vi "Get Plot at Mouse Click in Legend.vi"(0 "LegNumRows":u32, 5 "Legend:Position":T2, 7 "Legend:Size":T1, 9 "LegScrollPos":u32, 11 "Error In":errorcluster, 12 "Mouse Click Coordinates":cluster{"Horizontal":dbl, "Vertical":dbl}) -> (4 "Click is in Legend?":bool, 8 "Plot Index":i32, 15 "Error Out":errorcluster)   [LabVIEW 2019]
uses:
  <vilib>/Utility/miscctls.llb/LVPositionTypeDef.ctl
  <vilib>/Utility/miscctls.llb/LVBoundsTypeDef.ctl
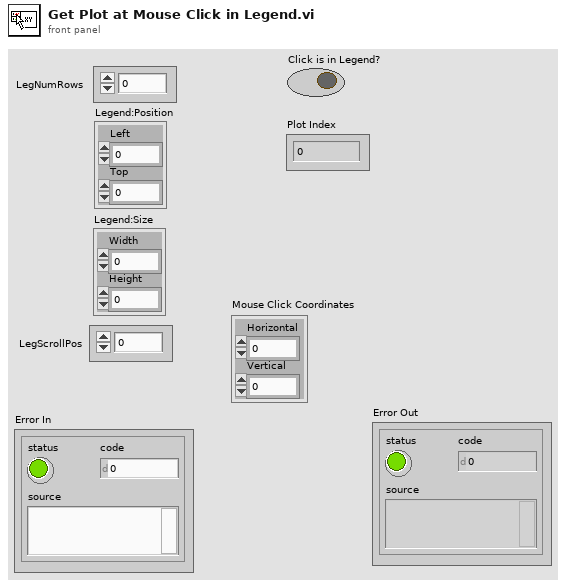
[diagram p1: front panel]
types:
  T1 = typedef "LVBoundsTypeDef.ctl" = cluster{"Width":u32, "Height":u32}
  T2 = typedef "LVPositionTypeDef.ctl" = cluster{"Left":i32, "Top":i32}
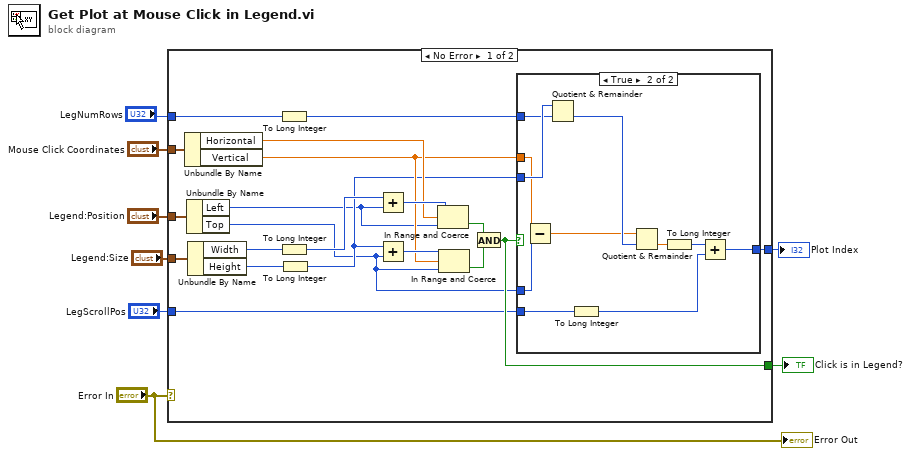
[diagram p0: block diagram]
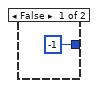
[diagram p2: hidden frame]
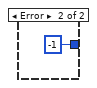
[diagram p3: hidden frame]
diagram:
  n1 = case shown="No Error" "Error In" {
    tunnel: "Mouse Click Coordinates" -> [w24 _]
    tunnel: "LegNumRows" -> [w22 _]
    tunnel: [w20 -1] -> w6
    tunnel: [w19 _] -> w5
    tunnel: "LegScrollPos" -> [w18 _]
    tunnel: "Legend:Position" -> [w14 _]
    tunnel: "Legend:Size" -> [w12 _]
    frame No Error {
      n2 = Unbundle By Name(w24) -> ("Horizontal"=w23:dbl, "Vertical"=w21:dbl)
      n3 = Unbundle By Name(w14) -> ("Left"=w9:i32, "Top"=w13:i32)
      n4 = Unbundle By Name(w12) -> ("Width"=w11:u32, "Height"=w10:u32)
      n5 = To Long Integer(number=w22) -> (32bit integer=w15:i32)
      n6 = To Long Integer(number=w11) -> (32bit integer=w17:i32)
      n7 = To Long Integer(number=w10) -> (32bit integer=w16:i32)
      n8 = Add(x=w17, y=w9) -> (x+y=w25:i32)
      n9 = Add(x=w16, y=w13) -> (x+y=w26:i32)
      n10 = In Range and Coerce(upper limit=w25, x=w23, lower limit=w9) -> (In Range?=w27:bool)  [unwired: 1 out]
      n11 = In Range and Coerce(upper limit=w26, x=w21, lower limit=w13) -> (In Range?=w28:bool)  [unwired: 1 out]
      n12 = And(x=w27, y=w28) -> (x .and. y?=w19:bool)
      n13 = case shown="True" w19 {
        tunnel: w16 -> [_ w40]
        tunnel: w15 -> [_ w39]
        tunnel: w13 -> [_ w34]
        tunnel: w21 -> [_ w35]
        tunnel: [-1 w32] -> w20
        tunnel: w18 -> [_ w31]
        frame False {
        }
        frame True {
          n14 = Subtract(x=w35, y=w34) -> (x-y=w33:dbl)
          n15 = Quotient & Remainder(x=w40, y=w39) -> (floor(x/y)=w38:i32)  [unwired: 1 out]
          n16 = To Long Integer(number=w31) -> (32bit integer=w30:i32)
          n17 = Quotient & Remainder(x=w33, y=w38) -> (floor(x/y)=w37:dbl)  [unwired: 1 out]
          n18 = To Long Integer(number=w37) -> (32bit integer=w36:i32)
          n19 = Add(x=w36, y=w30) -> (x+y=w32:i32)
        }
      }
    }
    frame Error {
    }
  }
  "Click is in Legend?" <- w5
  "Plot Index" <- w6
  "Error Out" <- "Error In"
